vi "Diagnostics.vi"(8 "error in (no error)":errorcluster, 10 "shutdown":refnum<user-event>, 11 "Modules":T3) -> (0 "Error 2":errorcluster)   [LabVIEW 2025]
uses:
  Libraries/USB IO/Classes/Hardware Selection.ctl
  Controls/Numeric Voltage.ctl
  <vilib>/Handler Framework/CmdQueue/Enqueue Single.vi
  <vilib>/Handler Framework/Handler Framework.lvlib
  Libraries/USB IO/USB IO.lvlib
  Libraries/Wheatstone Bridge/Wheatstone Bridge.lvlib
  Libraries/Motor/Motor.lvlib
panel:
  out "Angle":dbl format="%5.3f°"
  in  "Clear Motor Error":bool
  in  "Go To Angle":bool
  in  "CCW?":bool
  in  "Jog":bool
  in  "Speed [rpm]":dbl(slide)=9.818181818181818 min=0.0 max=100.0 scale=0.0..100.0
  in  "Angle":dbl(knob) scale=-90.0..90.0
  out "Voltage Chart 2":dbl(graph)
  out "Torque":dbl format="%5.3f lb-in"
  out "error out":errorcluster
  out "Voltage Chart":dbl(graph)
  in  "Digital Value":bool
  in  "Write":bool
  out "Voltage":T1 format="%5.3f V"
  in  "Read":bool
  in  "Lines":u16(ring) items=["Dev4/ai0", "Dev4/ai1", "Dev4/ai2", "Dev4/ai3", "Dev4/ai4", "Dev4/ai5", "Dev4/ai6", "Dev4/ai7", "Dev4/port0/line0", "Dev4/port0/line1", "Dev4/port0/line2", "Dev4/port0/line3"]
  in  "I/O Reconnect":bool
  in  "Serial Port":refnum<visa-resource-name>="N/A"
  in  "I/O Device":T2=enum."USB-6000"
  out "Module Names":string[](array[string])
  out "Error":errorcluster
  # "Diagnostics"
  # "Modules"
  # "USB I/O"
  # "TORQUE TRANSDUCER"
  # "MOTOR"
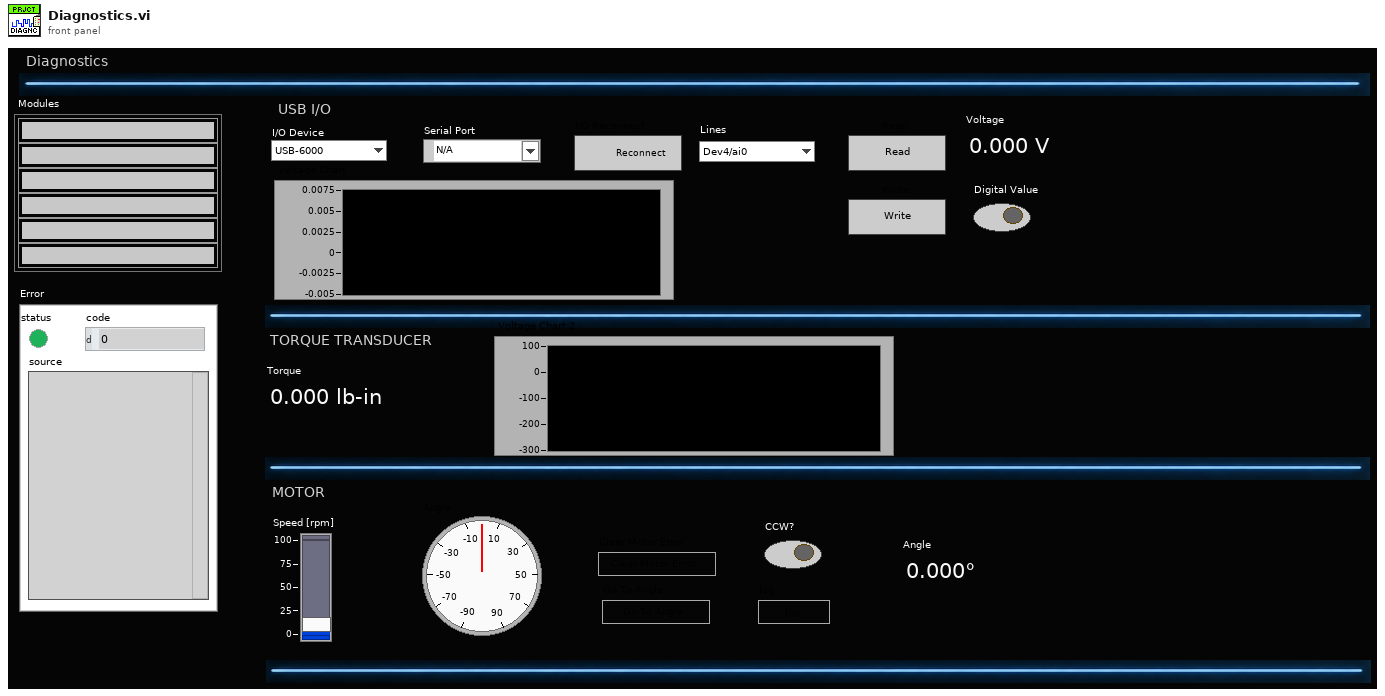
[diagram p1: front panel]
types:
  T1 = typedef "Numeric Voltage.ctl" = dbl
  T2 = typedef "Hardware Selection.ctl" = enum16{"Simulation", "USB-6000", "USB-6001", "Arduino Uno"}
  T3 = cluster{"Module IDs":i32[], "Module Names":string[]}
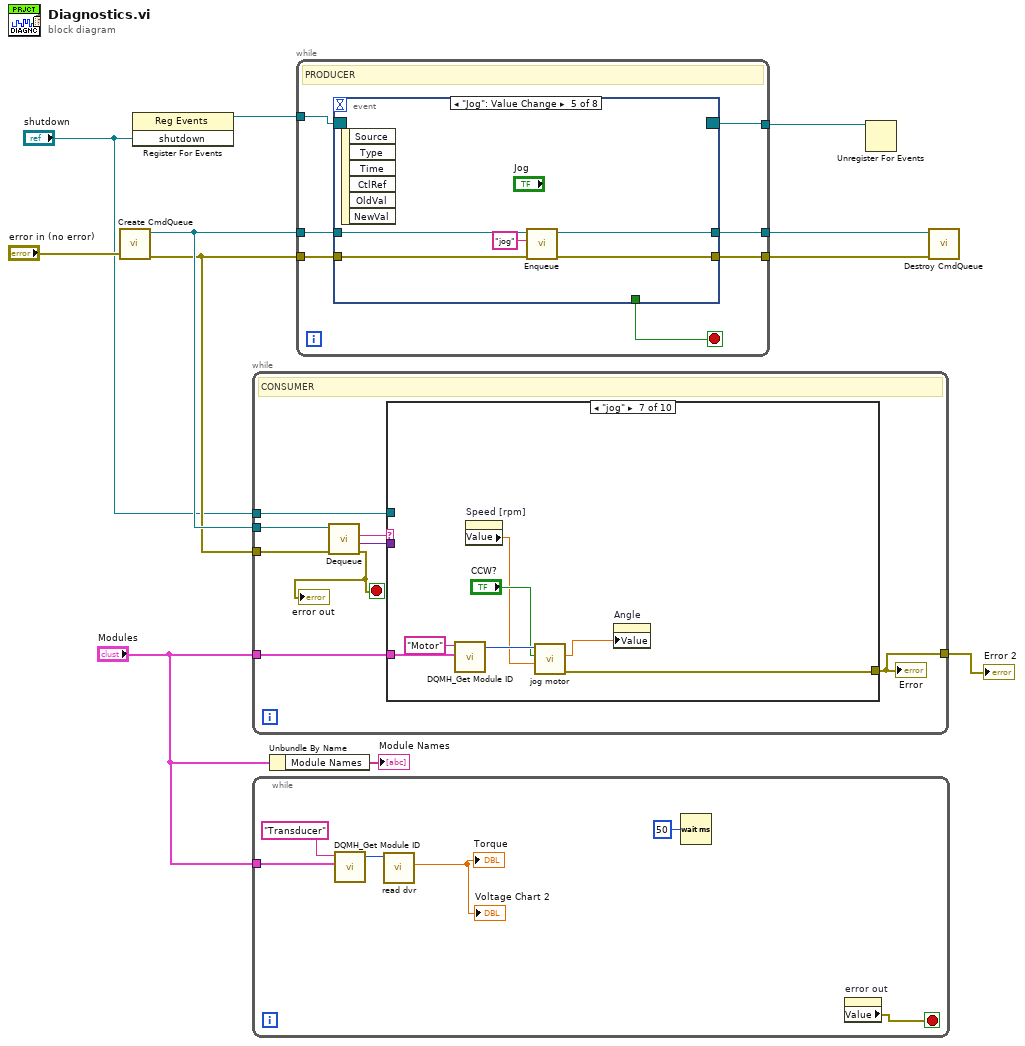
[diagram p0: block diagram]
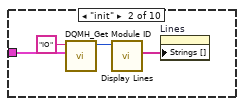
[diagram p3: hidden frame]
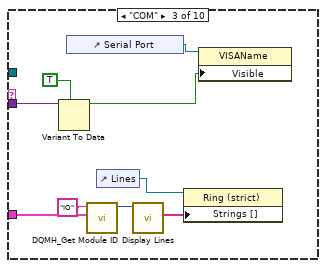
[diagram p4: hidden frame]
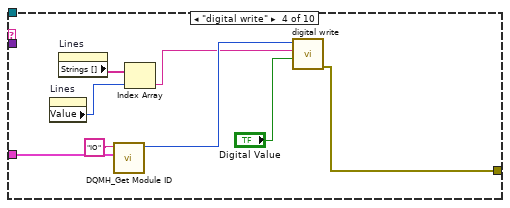
[diagram p5: hidden frame]
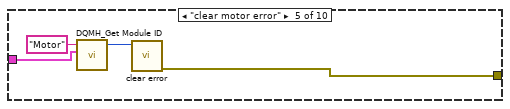
[diagram p6: hidden frame]
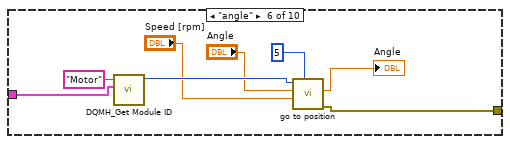
[diagram p7: hidden frame]
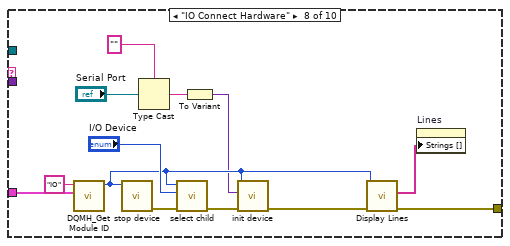
[diagram p8: hidden frame]
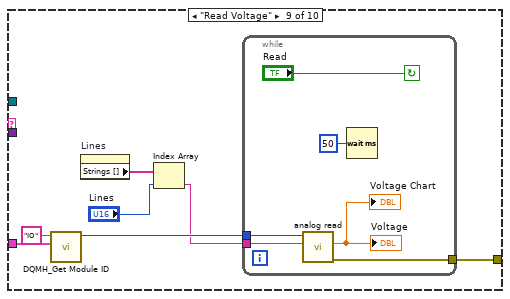
[diagram p9: hidden frame]
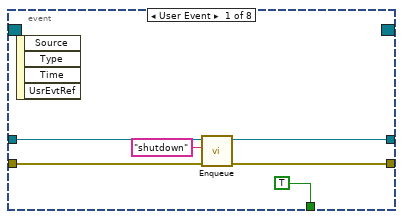
[diagram p11: hidden frame]
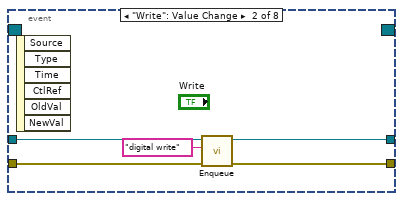
[diagram p12: hidden frame]
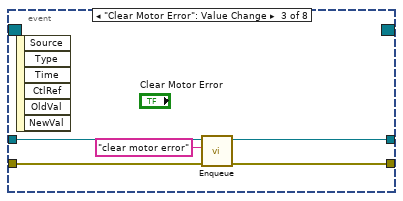
[diagram p13: hidden frame]
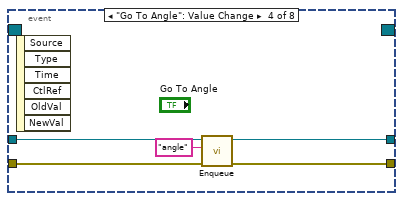
[diagram p14: hidden frame]
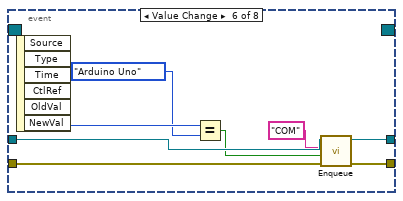
[diagram p15: hidden frame]
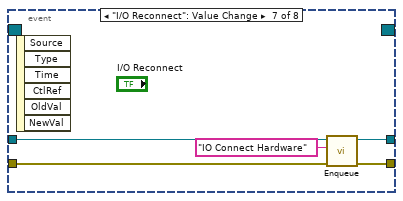
[diagram p16: hidden frame]
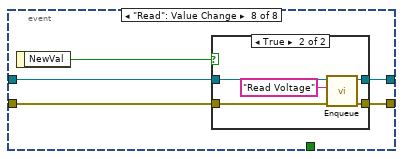
[diagram p17: hidden frame]
diagram:
  n1 = call <vilib>:"Create CmdQueue.vi"("error in (no error)"="error in (no error)") -> ("error out"=w8:errorcluster, "CmdQueue out"=w9:refnum<queue>)  [unwired: 9 in]
  n2 = register-events("shutdown") -> (reference out=w7:refnum<event-registration>)  [unwired: 2 in, 1 out]
  n3 = while {
    tunnel: w9 -> [w19]
    tunnel: w8 -> [w15]
    tunnel: "shutdown" -> [w14]
    tunnel: "Modules" -> [w13]
    tunnel: [w12] -> w2
    stop <- w16 stop-if-true
    # "CONSUMER"
    n4 = call <vilib>:"Dequeue.vi"("error in (no error)"=w15, "CmdQueue in"=w19) -> ("error out"=w16:errorcluster, "value"=w17:variant, "cmd"=w18:string)  [unwired: 5 in, 2 out]
    "error out" <- w16
    n5 = case shown="\"jog\"" w18 {
      tunnel: w17 -> [_ _ w31 _ _ _ _ _ _ _]
      tunnel: w14 -> [_ _ _ _ _ _ _ _ _ _]
      tunnel: w13 -> [_ w23 w25 w39 w43 w51 w59 w72 w79 _]
      tunnel: [_ _ _ w33 w41 w47 w54 w60 w73 _] -> w12
      frame "False", Default {
      }
      frame "init" {
        n6 = call "DQMH_Get Module ID.vi"("Modules"=w23, "Module Name"="IO") -> ("Module ID out"=w21:i32)  [unwired: 9 in]
        n7 = call "Display Lines.vi"("Module ID"=w21) -> ("Lines"=w20:string[])  [unwired: 7 in, 3 out]
        n8 = property on="Lines" class="Ring (strict)"("Strings []"=w20) -> ()  [unwired: 2 in, 2 out]
      }
      frame "COM" {
        n9 = Variant To Data(type=TRUE, Variant=w31) -> (data=w29:bool)  [unwired: 1 in, 1 out]
        n10 = control-ref of="Serial Port"() -> (w32:refnum<vi>)
        n11 = call "DQMH_Get Module ID.vi"("Modules"=w25, "Module Name"="IO") -> ("Module ID out"=w27:i32)  [unwired: 9 in]
        n12 = control-ref of="Lines"() -> (w24:refnum<vi>)
        n13 = call "Display Lines.vi"("Module ID"=w27) -> ("Lines"=w26:string[])  [unwired: 7 in, 3 out]
        n14 = property on="Property Node" class="Ring (strict)"(reference=w24, "Strings []"=w26) -> ()  [unwired: 1 in, 2 out]
        n15 = property class="VISAName"(reference=w32, "Visible"=w29) -> ()  [unwired: 1 in, 2 out]
      }
      frame "digital write" {
        n16 = property on="Lines" class="Ring (strict)"() -> ("Value"=w35:u16)  [unwired: 2 in, 2 out]
        n17 = property on="Lines" class="Ring (strict)"() -> ("Strings []"=w36:string[])  [unwired: 2 in, 2 out]
        n18 = call "DQMH_Get Module ID.vi"("Modules"=w39, "Module Name"="IO") -> ("Module ID out"=w38:i32)  [unwired: 9 in]
        n19 = Index Array(array=w36, index=w35) -> (element=w34:string)
        n20 = call "digital write.vi"("On/Off"="Digital Value", "Line"=w34, "Module ID"=w38) -> ("error out"=w33:errorcluster)  [unwired: 7 in, 1 out]
      }
      frame "clear motor error" {
        n21 = call "DQMH_Get Module ID.vi"("Modules"=w43, "Module Name"="Motor") -> ("Module ID out"=w42:i32)  [unwired: 9 in]
        n22 = call "clear error.vi"("Module ID"=w42) -> ("error out"=w41:errorcluster)  [unwired: 9 in, 1 out]
      }
      frame "angle" {
        n23 = call "DQMH_Get Module ID.vi"("Modules"=w51, "Module Name"="Motor") -> ("Module ID out"=w50:i32)  [unwired: 9 in]
        n24 = call "go to position.vi"("Pause Time [ms]"=5, "Velocity [rpm]"="Speed [rpm]", "Position"="Angle", "Module ID"=w50) -> ("error out"=w47:errorcluster, "Position 2"=→"Angle":dbl)  [unwired: 5 in, 1 out]
      }
      frame "jog" {
        n25 = call "DQMH_Get Module ID.vi"("Modules"=w59, "Module Name"="Motor") -> ("Module ID out"=w57:i32)  [unwired: 9 in]
        n26 = property on="Speed [rpm]" class="Slide (strict)"() -> ("Value"=w55:dbl)  [unwired: 2 in, 2 out]
        n27 = call "jog motor.vi"("Speed [rpm]"=w55, "CCW? (T)"="CCW?", "Module ID"=w57) -> ("error out"=w54:errorcluster, "Position"=w53:dbl)  [unwired: 6 in, 1 out]
        n28 = property on="Angle" class="DigNum (strict)"("Value"=w53) -> ()  [unwired: 2 in, 2 out]
      }
      frame "IO Connect Hardware" {
        n29 = call "DQMH_Get Module ID.vi"("Modules"=w72, "Module Name"="IO") -> ("Module ID out"=w69:i32)  [unwired: 9 in]
        n30 = call "stop device.vi"("Module ID"=w69) -> ("error out"=w63:errorcluster)  [unwired: 9 in, 1 out]
        n31 = Type Cast(type="", x="Serial Port") -> (*(type *) &x=w65:string)
        n32 = call "select child.vi"("error in"=w63, "Hardware"="I/O Device", "Module ID"=w69) -> ("error out"=w61:errorcluster)  [unwired: 7 in, 1 out]
        n33 = To Variant(anything=w65) -> (Variant=w64:variant)
        n34 = call "init device.vi"("error in"=w61, "Variant"=w64, "Module ID"=w69) -> ("error out"=w62:errorcluster)  [unwired: 7 in, 1 out]
        n35 = call "Display Lines.vi"("error in"=w62, "Module ID"=w69) -> ("error out"=w60:errorcluster, "Lines"=w68:string[])  [unwired: 6 in, 2 out]
        n36 = property on="Lines" class="Ring (strict)"("Strings []"=w68) -> ()  [unwired: 2 in, 2 out]
      }
      frame "Read Voltage" {
        n37 = call "DQMH_Get Module ID.vi"("Modules"=w79, "Module Name"="IO") -> ("Module ID out"=w77:i32)  [unwired: 9 in]
        n38 = property on="Lines" class="Ring (strict)"() -> ("Strings []"=w76:string[])  [unwired: 2 in, 2 out]
        n39 = Index Array(array=w76, index="Lines") -> (element=w74:string)
        n40 = while {
          tunnel: w77 -> [w85]
          tunnel: w74 -> [w84]
          tunnel: [w83] -> w73
          stop <- "Read" continue-if-true
          n41 = call "analog read.vi"("Line"=w84, "Module ID"=w85) -> ("error out"=w83:errorcluster, "Voltage"=→"Voltage" →"Voltage Chart":T1)  [unwired: 7 in, 1 out]
          n42 = Wait (ms)(milliseconds to wait=u32 50) -> ()  [unwired: 1 out]
        }
      }
      frame "shutdown" {
      }
    }
    "Error" <- w12
  }
  "Error 2" <- w2
  n43 = while {
    tunnel: "Modules" -> [w91]
    stop <- w88 stop-if-true
    n44 = call "DQMH_Get Module ID.vi"("Modules"=w91, "Module Name"="Transducer") -> ("Module ID out"=w89:i32)  [unwired: 9 in]
    n45 = call "read dvr.vi"("Module ID"=w89) -> ("Numeric"=→"Voltage Chart 2" →"Torque":dbl)  [unwired: 8 in, 2 out]
    n46 = Wait (ms)(milliseconds to wait=u32 50) -> ()  [unwired: 1 out]
    n47 = property on="error out" class="Clust (strict)"() -> ("Value"=w88:errorcluster)  [unwired: 2 in, 2 out]
  }
  n48 = Unbundle By Name("Modules") -> ("Module Names"=→"Module Names":string[])
  n49 = while {
    tunnel: w9 -> [w98]
    tunnel: [w97] -> w11
    tunnel: w8 -> [w96]
    tunnel: [w95] -> w10
    tunnel: w7 -> [w93]
    tunnel: [w92] -> w6
    stop <- w94 stop-if-true
    # "PRODUCER"
    n50 = event shown="[4] \"Jog\": Value Change" {
      selector: w93 -> [_ _ _ _ _ _ _ _]
      dyn-events: [_ _ _ _ _ _ _ _] -> w92
      timeout: _ -> [_ _ _ _ _ _ _ _]
      tunnel: w98 -> [w104 w109 w114 w119 w124 w128 w135 w140]
      tunnel: [w103 w108 w113 w118 w123 w129 w136 w141] -> w97
      tunnel: w96 -> [w102 w107 w112 w117 w122 w127 w134 w139]
      tunnel: [w101 w106 w111 w116 w121 w130 w137 w142] -> w95
      tunnel: [TRUE ("Discard?") _ _ _ _ _ _ _] -> w94
      event User Event {
        n51 = event-data() -> ()  [unwired: 1 in, 4 out]
        n52 = call-poly <vilib>:"Enqueue.vi"("error in (no error)"=w102, "Command"="shutdown", "CmdQueue in"=w104) -> ("error out"=w101:errorcluster, "CmdQueue out"=w103:refnum<queue>)  [unwired: 7 in]
      }
      event "Write": Value Change {
        n53 = event-data() -> ()  [unwired: 1 in, 6 out]
        n54 = call-poly <vilib>:"Enqueue.vi"("error in (no error)"=w107, "Command"="digital write", "CmdQueue in"=w109) -> ("error out"=w106:errorcluster, "CmdQueue out"=w108:refnum<queue>)  [unwired: 7 in]
      }
      event "Clear Motor Error": Value Change {
        n55 = event-data() -> ()  [unwired: 1 in, 6 out]
        n56 = call-poly <vilib>:"Enqueue.vi"("error in (no error)"=w112, "Command"="clear motor error", "CmdQueue in"=w114) -> ("error out"=w111:errorcluster, "CmdQueue out"=w113:refnum<queue>)  [unwired: 7 in]
      }
      event "Go To Angle": Value Change {
        n57 = event-data() -> ()  [unwired: 1 in, 6 out]
        n58 = call-poly <vilib>:"Enqueue.vi"("error in (no error)"=w117, "Command"="angle", "CmdQueue in"=w119) -> ("error out"=w116:errorcluster, "CmdQueue out"=w118:refnum<queue>)  [unwired: 7 in]
      }
      event "Jog": Value Change {
        n59 = event-data() -> ()  [unwired: 1 in, 6 out]
        n60 = call-poly <vilib>:"Enqueue.vi"("error in (no error)"=w122, "Command"="jog", "CmdQueue in"=w124) -> ("error out"=w121:errorcluster, "CmdQueue out"=w123:refnum<queue>)  [unwired: 7 in]
      }
      event Value Change {
        n61 = event-data() -> ("NewVal"=w132:T2)  [unwired: 1 in, 5 out]
        n62 = Equal?(x=w132, y=Hardware_Selection."Arduino Uno" ("NewVal")) -> (x = y?=w125:bool)
        n63 = call-poly <vilib>:"Enqueue.vi"("error in (no error)"=w127, "Value"=w125, "Command"="COM", "CmdQueue in"=w128) -> ("error out"=w130:errorcluster, "CmdQueue out"=w129:refnum<queue>)  [unwired: 6 in]
      }
      event "I/O Reconnect": Value Change {
        n64 = event-data() -> ()  [unwired: 1 in, 6 out]
        n65 = call-poly <vilib>:"Enqueue.vi"("error in (no error)"=w134, "Command"="IO Connect Hardware", "CmdQueue in"=w135) -> ("error out"=w137:errorcluster, "CmdQueue out"=w136:refnum<queue>)  [unwired: 7 in]
      }
      event "Read": Value Change {
        n66 = event-data() -> ("NewVal"=w138:bool)  [unwired: 1 in]
        n67 = case shown="True" w138 {
          tunnel: [w143 w149] -> w142
          tunnel: [w144 w148] -> w141
          tunnel: w140 -> [w144 w147]
          tunnel: w139 -> [w143 w146]
          frame False {
          }
          frame True {
            n68 = call-poly <vilib>:"Enqueue.vi"("error in (no error)"=w146, "Command"="Read Voltage", "CmdQueue in"=w147) -> ("error out"=w149:errorcluster, "CmdQueue out"=w148:refnum<queue>)  [unwired: 7 in]
          }
        }
      }
    }
  }
  n69 = Unregister For Events(event registration refnum=w6) -> ()  [unwired: 1 in, 1 out]
  n70 = call <vilib>:"Destroy CmdQueue.vi"("error in (no error)"=w10, "CmdQueue in"=w11) -> ()  [unwired: 9 in, 1 out]
